vi "Counter.vi"() -> ()   [LabVIEW 2018]
uses:
  <vilib>/Instr/_visa.llb/VISA Configure Serial Port (Instr).vi
panel:
  out "Waveform Chart":T1(graph)
  in  "Trigger Mode":u16(ring) items=["TTL", "NIM"]
  in  "Config SET":bool
  in  "Counter Mode":u16(ring) items=["Single", "Pairs"]
  in  "Gate Timing":dbl
  in  "Max Read Buffer":i32=100
  in  "stop":bool
  out "Return Text":string
  in  "Serial Settings":T2={"baud rate"=115200, "data bits"=8, "parity"=enum."None", "stop bits"=10, "flow control"=2} {"flow control" items=["None"=0, "XON/XOFF"=1, "RTS/CTS"=2, "DTR/DSR"=4]; "stop bits" items=["1.0"=10, "1.5"=15, "2.0"=20]; "data bits" min=5 max=8 step=1; "baud rate" items=["75"=75, "110"=110, "134"=134, "150"=150, "300"=300, "600"=600, "1200"=1200, "1800"=1800, "2400"=2400, "4800"=4800, "7200"=7200, "4"=9600, "14400"=14400, "19200"=19200, "28800"=28800, "38400"=38400, "56000"=56000, "57600"=57600, "115200"=115200, "128000"=128000, "230400"=230400]}
  in  "VISA resource name":refnum<visa-resource-name>="COM1"
  # "Simple counter VI for continuous probing of counter values, when initializing this VI :\n1) Make sure the correct COM is selected or it will return NULL strings.\n2) Config SET button MUST be TRUE at start of program to ensure the device is \ninitialized properly with the required gate timing, counter mode and trigger mode.\n\nDuring operation you can change settings (Gate Timing, Counter Mode, Trigger Mode), \npress Config SET once to commit change."
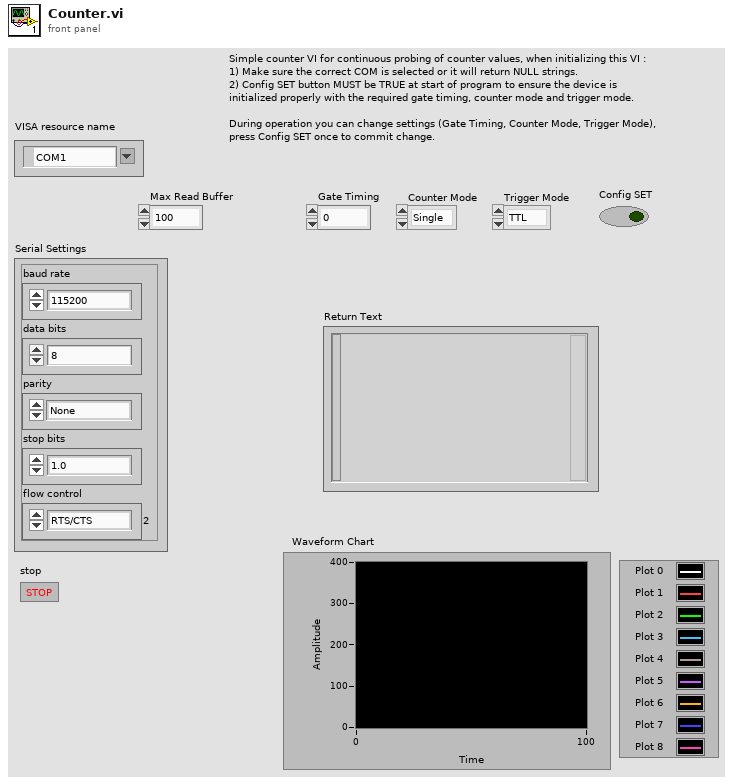
[diagram p1: front panel]
types:
  T1 = cluster{"[0]":dbl, "[1]":dbl, "[2]":dbl, "[3]":dbl, "[4]":dbl, "[5]":dbl, "[6]":dbl, "[7]":dbl, "[8]":dbl}
  T2 = cluster{"baud rate":u32, "data bits":u16, "parity":enum16{"None", "Odd", "Even", "Mark", "Space"}, "stop bits":u16, "flow control":u16}
  T3 = cluster{"array type (2D Dbl)[0]":dbl, "array type (2D Dbl)[1]":dbl, "array type (2D Dbl)[2]":dbl, "array type (2D Dbl)[3]":dbl, "array type (2D Dbl)[4]":dbl, "array type (2D Dbl)[5]":dbl, "array type (2D Dbl)[6]":dbl, "array type (2D Dbl)[7]":dbl, "array type (2D Dbl)[8]":dbl}
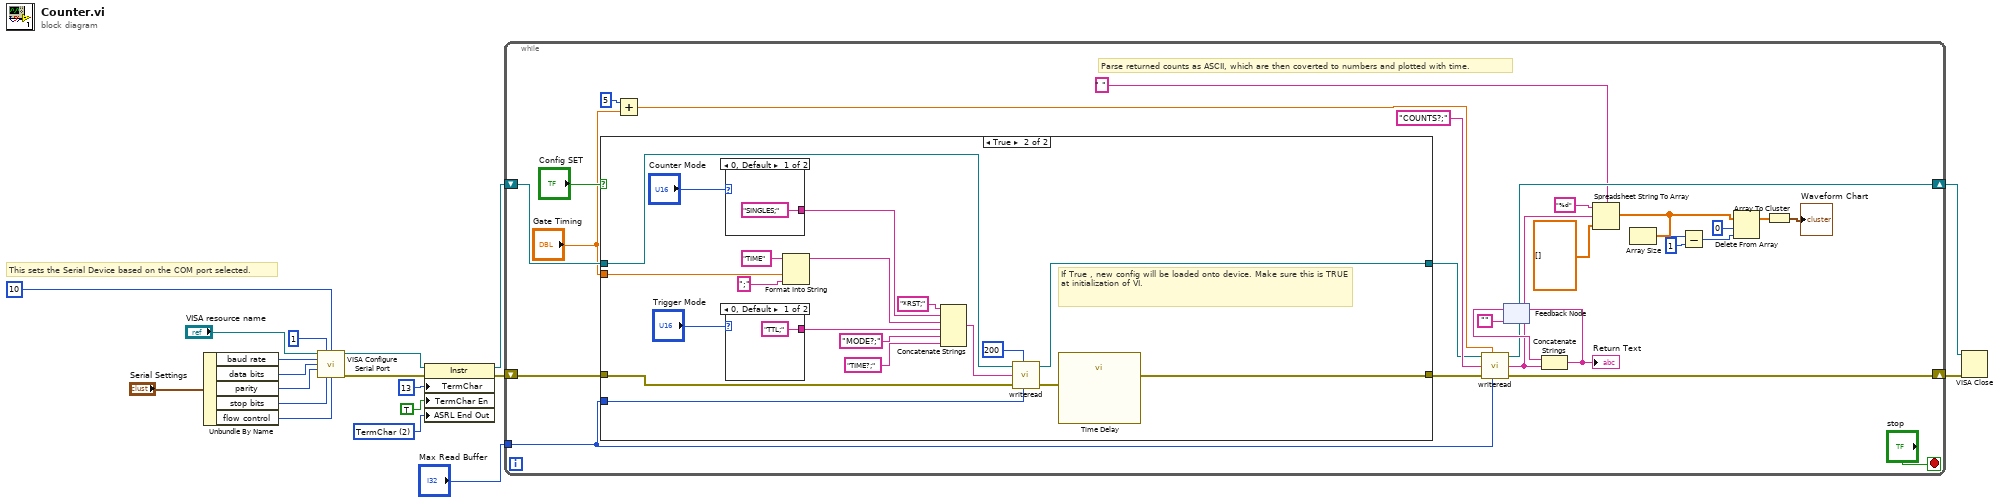
[diagram p0: block diagram]
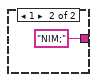
[diagram p3: hidden frame]
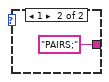
[diagram p4: hidden frame]
diagram:
  w1 = u16 2 items=["None", "Last Bit", "TermChar", "Break"] ("Serial Settings:End Mode for Writes")
  # "This sets the Serial Device based on the COM port selected."
  n1 = Unbundle By Name("Serial Settings") -> ("baud rate"=w17:u32, "data bits"=w16:u16, "parity"=w15:enum16{"None", "Odd", "Even", "Mark", "Space"}, "stop bits"=w14:u16, "flow control"=w13:u16)
  n2 = call-poly "VISA Configure Serial Port"("VISA resource name"="VISA resource name", "timeout (10sec)"=1, "termination char\n(0xA = '\\n' = LF)"=10, "baud rate (9600)"=w17, "data bits (8)"=w16, "parity (0:none)"=w15, "stop bits (10: 1 bit)"=w14, "flow control (0:none)"=w13) -> ("VISA resource name out"=w7:refnum<visa-resource-name>, "error out"=w5:errorcluster)  [unwired: 2 in, 4 out]
  n3 = property class="Instr"(reference=w7, error in=w5, "TermChar"=13, "TermChar En"=TRUE, "ASRL End Out"=w1) -> (reference out=w6:refnum<visa-resource-name>, error out=w4:errorcluster)
  n4 = while {
    shift-right: [w41] -> w9
    shift-left: w4 -> [w35]
    shift-right: [w42] -> w10
    shift-left: w6 -> [w36]
    tunnel: "Max Read Buffer" -> [w34]
    stop <- "stop" stop-if-true
    # "Parse returned counts as ASCII, which are then coverted to numbers and plotted with time."
    n5 = case shown="True" "Config SET" {
      tunnel: [w48 w63] -> w38
      tunnel: [w47 w61] -> w37
      tunnel: w36 -> [w48 w67]
      tunnel: w35 -> [w47 w66]
      tunnel: w34 -> [_ w64]
      tunnel: "Gate Timing" -> [_ w54]
      frame False {
      }
      frame True {
        # "If True , new config will be loaded onto device. Make sure this is TRUE at initialization of VI."
        n6 = case shown="0, Default" "Counter Mode" {
          tunnel: ["SINGLES;" "PAIRS;"] -> w59
          frame 0, Default {
          }
          frame 1 {
          }
        }
        n7 = case shown="0, Default" "Trigger Mode" {
          tunnel: ["TTL;" "NIM;"] -> w51
          frame 0, Default {
          }
          frame 1 {
          }
        }
        n8 = Format Into String(initial string="TIME", w54, ";") -> (resulting string=w60:string)  [unwired: 2 in, 1 out]
        n9 = Concatenate Strings("*RST;", w59, w60, w51, "MODE?;", "TIME?;") -> (w53:string)
        n10 = call "writeread.vi"("VISA resource input"=w67, "Read Delay"=200, "write buffer"=w53, "error in (no error)"=w66, "Max Read Buffer"=w64) -> ("VISA resource out"=w63:refnum<visa-resource-name>, "error out"=w62:errorcluster)  [unwired: 2 in, 1 out]
        n11 = call "Time Delay"("error in (no error)"=w62) -> ("error out"=w61:errorcluster)  [unwired: 10 in]
      }
    }
    n12 = Add(x=5, y="Gate Timing") -> (x+y=w20:dbl)
    n13 = call "writeread.vi"("VISA resource input"=w38, "Read Delay"=w20, "write buffer"="COUNTS?;", "error in (no error)"=w37, "Max Read Buffer"=w34) -> ("VISA resource out"=w42:refnum<visa-resource-name>, "Response 2"=w33:string, "error out"=w41:errorcluster)  [unwired: 2 in]
    n14 = feedback #1("") -> (w46:string)
    n15 = Concatenate Strings(w46, w33) -> (w44:string)
    "Return Text" <- w44
    n16 = feedback-in #1(w44) -> ()
    n17 = Spreadsheet String To Array(delimiter (Tab)=" ", format string="%d", spreadsheet string=w33, array type (2D Dbl)=dbl[] []) -> (array=w29:dbl[])
    n18 = Array Size(array=w29) -> (size(s)=w25:i32)
    n19 = Subtract(x=w25, y=1) -> (x-y=w24:i32)
    n20 = Delete From Array(array=w29, length=0, index=w24) -> (array with subset deleted=w27:dbl[])  [unwired: 1 out]
    n21 = Array To Cluster(array=w27) -> (cluster=→"Waveform Chart":T3)
  }
  n22 = VISA Close(VISA resource name=w10, error in (no error)=w9) -> ()  [unwired: 1 out]
